vi "JSON Routing Channel Template Tests.vi"(8 "error in":errorcluster) -> (0 "error out":errorcluster)   [LabVIEW 2020, in "Test_Routing Templates.lvlib"]
uses:
  Test_Routing Templates.lvlib
  <vilib>/addons/_JKI Toolkits/Caraya/classes/Test/Test.lvclass
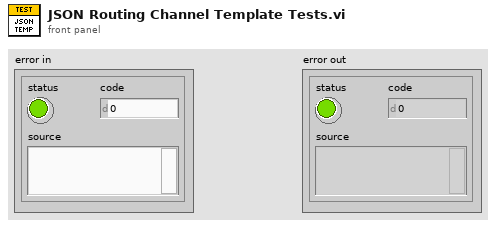
[diagram p1: front panel]
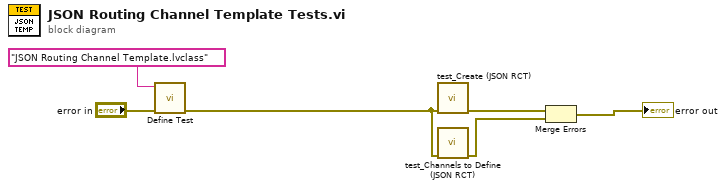
[diagram p0: block diagram]
diagram:
  n1 = call <vilib>:"Define Test.vi"("error in (no error)"="error in", "Label (VI Title)"="JSON Routing Channel Template.lvclass") -> ("error out"=w2:errorcluster)  [unwired: 9 in]
  n2 = call "test_Create (JSON RCT).vi"("error in"=w2) -> ("error out"=w4:errorcluster)  [unwired: 10 in]
  n3 = call "test_Channels to Define (JSON RCT).vi"("error in"=w2) -> ("error out"=w1:errorcluster)  [unwired: 10 in]
  n4 = Merge Errors(w4, w1) -> (→"error out":errorcluster)
